vi "random.vi"(1 "输入值":dbl, 2 "lower bound (0)":dbl caption="下限(0)", 3 "布尔":bool, 4 "upper bound (100)":dbl=100.0 caption="上限(100)") -> (0 "number":dbl caption="输出值")   [LabVIEW 2020]
uses:
  <vilib>/numeric/Random Number (Range) DBL.vi
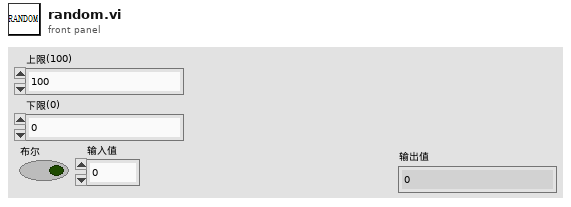
[diagram p1: front panel]
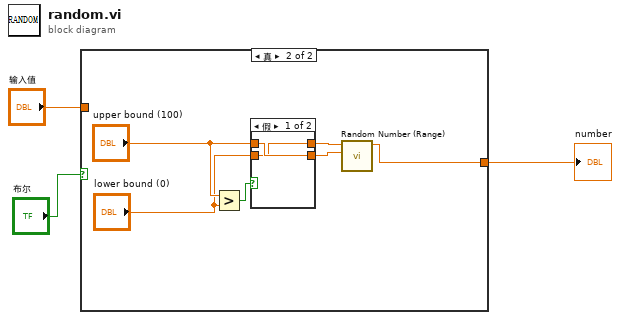
[diagram p0: block diagram]
diagram:
  n1 = case shown="真" "布尔" {
    tunnel: [w4 w5] -> w2
    tunnel: "输入值" -> [w4 _]
    frame False {
    }
    frame True {
      n2 = Greater?(x="upper bound (100)", y="lower bound (0)") -> (0:w10:bool)
      n3 = case shown="假" w10 {
        tunnel: [w11 w14] -> w9
        tunnel: "upper bound (100)" -> [w12 w14]
        tunnel: [w12 w13] -> w7
        tunnel: "lower bound (0)" -> [w11 w13]
        frame False {
        }
        frame True {
        }
      }
      n4 = call-poly <vilib>:"Random Number (Range).vi"("lower bound (0)"=w7, "upper bound (100)"=w9) -> ("number"=w5:dbl)  [unwired: 9 in]
    }
  }
  "number" <- w2
